vi "GetTensionPosofEachCycle.vi"(8 "error in (no error)":errorcluster, 11 "CAlexData2 in":refnum<class "CAlex2_Data.lvclass">) -> (0 "error out":errorcluster, 1 "VarColHeaders":string[](array[string]), 2 "AnklePosEachCycle":dbl[][][](array[numeric]), 3 "CAlexData2 out":refnum<class "CAlex2_Data.lvclass">)   [LabVIEW 2016, in "CAlex2_Data.lvclass"]
uses:
  CAlex2_Data.lvclass
  C:/Users/randh/Desktop/BILATERAL/CAlex2-controller/Sim&Process/DataProcess/ExpData/ExpData.lvclass
  ExpData/ExpData.lvclass
  <vilib>/AuZn/auzn custom VIs/AuZnCustomVI.lvlib
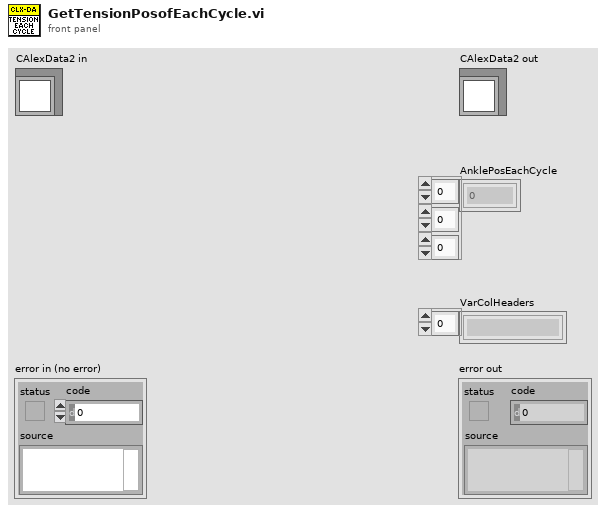
[diagram p1: front panel]
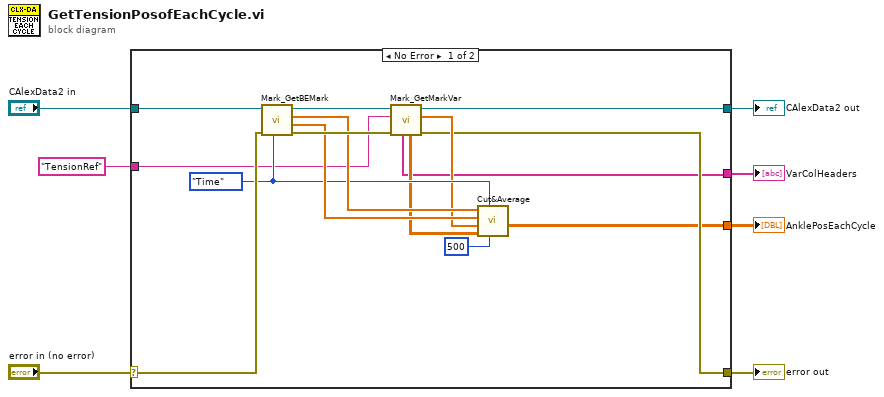
[diagram p0: block diagram]
diagram:
  n1 = case shown="No Error" "error in (no error)" {
    selector: "error in (no error)" -> [w21 w24]
    tunnel: [w12 w24] -> w6
    tunnel: [w19 w23] -> w4
    tunnel: "CAlexData2 in" -> [w22 w23]
    tunnel: [w10 _] -> w3
    tunnel: "TensionRef" ("Name") -> [w11 _]
    tunnel: [w9 _] -> w1
    frame No Error {
      w15 = enum16{"Time", "Percentage", "Index"}."Time" ("Type (Time)")
      n2 = call "Mark_GetBEMark.vi"("Type (Time)"=w15, "error in (no error)"=w21, "ExpData In"=w22) -> ("error out"=w18:errorcluster, "End"=w16:dbl[], "Begin"=w17:dbl[], "ExpData Out"=w20:refnum<class "CAlex2_Data.lvclass">)  [unwired: 4 in, 1 out]
      n3 = call "Mark_GetMarkVar.vi"("error in (no error)"=w18, "VarName"=w11, "ExpData in"=w20) -> ("error out"=w12:errorcluster, "Time"=w13:dbl[], "ExpData out"=w19:refnum<class "CAlex2_Data.lvclass">, "MarkVar_All"=w14:dbl[][], "VarColHeaders"=w9:string[])  [unwired: 3 in, 1 out]
      n4 = call <vilib>:"Cut&Average.vi"("Dilate Length (200)"=500, "Input Type (Time)"=w15, "Data"=w14, "Time"=w13, "End"=w16, "Begin"=w17) -> ("Dilated"=w10:dbl[][][])  [unwired: 5 out]
    }
    frame Error {
    }
  }
  "error out" <- w6
  "CAlexData2 out" <- w4
  "AnklePosEachCycle" <- w3
  "VarColHeaders" <- w1
